vi "InitializeMotorStage.vi"(8 "params":T3 {"Update Flags" format="%.0x"; "Goal Type" items=["Unlimited", "Distance", "Time", "Stop"]; "RunState" format="%02.0f" items=["IDLE"=0, "RAMPUP"=16, "RUNNING"=32, "RAMPDOWN"=64]; "RegMode" format="%02.0f" items=["IDLE", "SPEED", "SYNC"]; "Mode" format="%.0x"}, 9 "Port":T2 items=["Port A", "Port B", "Port C"]) -> ()   [LabVIEW 2009]
uses:
  MotorStageDefinition.ctl
  Move/RegMode.ctl
  Move/RunState.ctl
  <vilib>/NXT/Block Support/NXT_OutputGoalType.ctl
  <vilib>/NXT/Block Support/NXT_OutputPort.ctl
  NXTOutputRefnum.ctl
  Program Files/National Instruments/LabVIEW 2009/resource/objmgr/NXTInputOutput.rc
panel:
  in  "Generic Refnum Name":T1
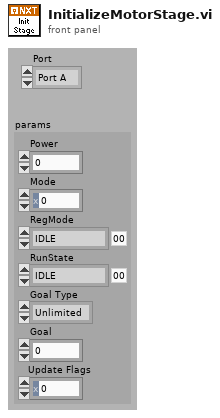
[diagram p1: front panel]
types:
  T1 = typedef "NXTOutputRefnum.ctl" = refnum<k21>
  T2 = typedef "NXT_OutputPort.ctl" = u8
  T3 = typedef "MotorStageDefinition.ctl" = cluster{"Power":i8, "Mode":u8, "RegMode":T4, "RunState":T5, "Goal Type":T6, "Goal":u32, "Update Flags":u8}
  T4 = typedef "RegMode.ctl" = u8
  T5 = typedef "RunState.ctl" = u8
  T6 = typedef "NXT_OutputGoalType.ctl" = u16
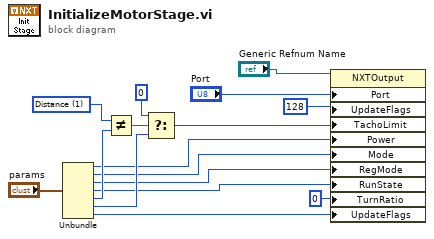
[diagram p0: block diagram]
diagram:
  w11 = T6 1 items=["Unlimited", "Distance", "Time", "Stop"] ("x")
  n1 = Unbundle("params") -> ("Power"=w7:i8, "Mode"=w3:u8, "RegMode"=w5:T4, "RunState"=w6:T5, "Goal Type"=w9:T6, "Goal"=w8:u32, "Update Flags"=w4:u8)
  n2 = Not Equal?(x=w11, y=w9) -> (x != y?=w13:bool)
  n3 = Select(t=u32 0, s=w13, f=w8) -> (s? t:f=w10:u32)
  n4 = property class="NXTOutput"(reference="Generic Refnum Name", "Port"="Port", "UpdateFlags"=u8 128 ("Port"), "TachoLimit"=w10, "Power"=w7, "Mode"=w3, "RegMode"=w5, "RunState"=w6, "TurnRatio"=i8 0, "UpdateFlags"=w4) -> ()  [unwired: 1 in, 2 out]
